vi "Qualify Library Icon Core.vi"(0 "VI Reference":refnum<vi>, 11 "error in":errorcluster) -> (3 "Class?":bool, 4 "Good Library Icon":bool, 6 "Maximum Number of Rows":i32, 8 "Library Path":path, 10 "Number of Rows in Icon":i32, 14 "Icon Image":picture, 15 "error out":errorcluster)   [LabVIEW 2025, in "Text-Based VI Icon.lvlib"]
uses:
  <vilib>/LabVIEW Icon API/Set Text Icon/Text-Based VI Icon.lvlib
panel:
  out "Left and Right Good (for Debugging)":bool
  out "Top and Bottom Good (for Debugging)":bool
  out "Good Frame Color (for Debugging)":bool
  out "Supported Size or Shape (for Debugging)":bool
  out "Last True Mask + 1 (for Debugging)":i32
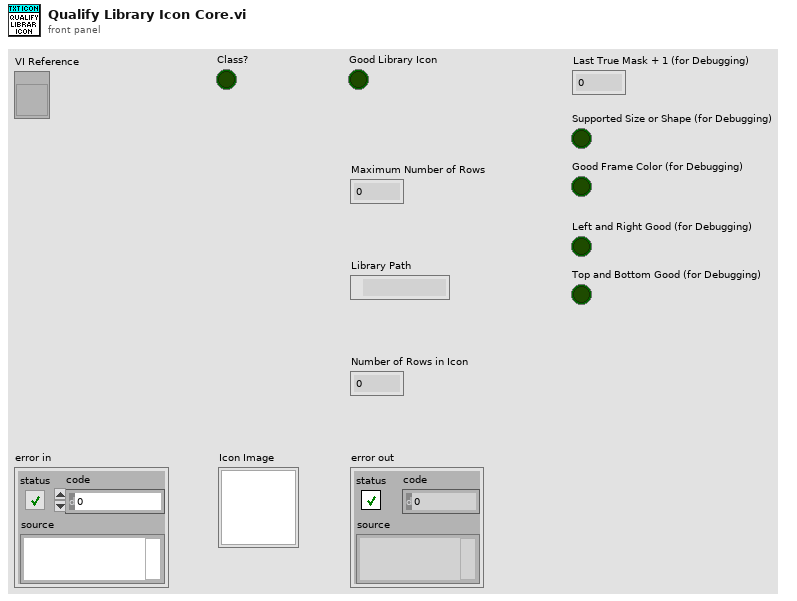
[diagram p1: front panel]
types:
  T1 = typedef "imagedata.ctl" = cluster{"image type":i32, "image depth":i32, "image":u8[], "mask":u8[], "colors":u32[], "Rectangle":cluster{"left":i16, "top":i16, "right":i16, "bottom":i16}}
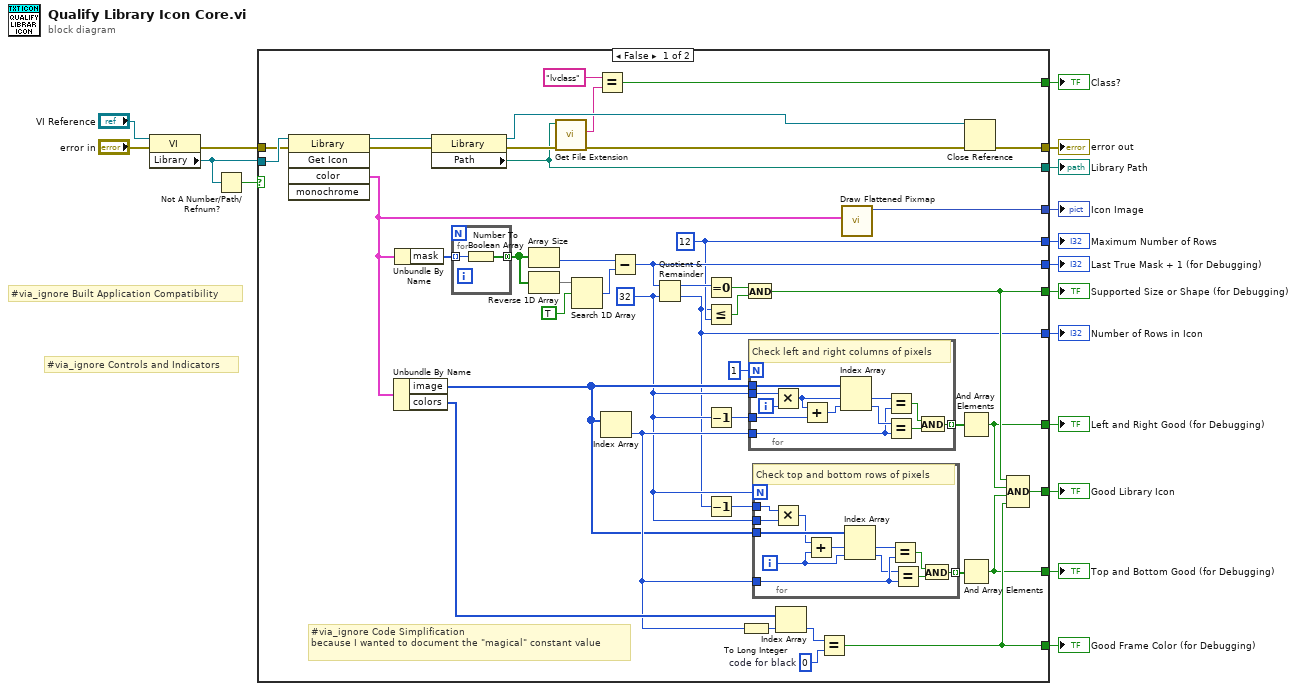
[diagram p0: block diagram]
diagram:
  # "#via_ignore Built Application Compatibility"
  # "#via_ignore Controls and Indicators"
  n1 = property class="VI"(reference="VI Reference", error in="error in") -> (error out=w15:errorcluster, "Library"=w16:refnum<vi>)  [unwired: 1 out]
  n2 = Not A Number/Path/Refnum?(number/path/refnum=w16) -> (NaN/Path/Refnum?=w17:bool)
  n3 = case shown="False" w17 {
    tunnel: w16 -> [w60 _]
    tunnel: w15 -> [w59 w87]
    tunnel: [w28 w87] -> w14
    tunnel: [w49 _] -> w13
    tunnel: [w36 _] -> w12
    tunnel: [w34 _] -> w11
    tunnel: [w33 _] -> w10
    tunnel: [w35 _] -> w9
    tunnel: [w37 _] -> w8
    tunnel: [w32 _] -> w7
    tunnel: [w21 _] -> w6
    tunnel: [w29 _] -> w3
    tunnel: [w22 _] -> w2
    tunnel: [w19 _] -> w1
    frame False {
      w47 = u32 0  # code for black
      w29 = 12 ("y")
      w38 = 32 ("y")
      # "#via_ignore Code Simplification\nbecause I wanted to document the \"magical\" constant value"
      n4 = invoke class="Library" method="Get Icon"(reference=w60, error in=w59) -> (reference out=w31:refnum<vi>, error out=w30:errorcluster, "color"=w20:T1)  [unwired: 3 in, 2 out]
      n5 = Unbundle By Name(w20) -> ("image"=w42:u8[], "colors"=w48:u32[])
      n6 = Unbundle By Name(w20) -> ("mask"=w55:u8[])
      n7 = property class="Library"(reference=w31, error in=w30) -> (reference out=w27:refnum<vi>, error out=w26:errorcluster, "Path"=w21:path)
      n8 = for {
        tunnel: w55 -> [w86] mode=indexing
        tunnel: [w85] -> w52 mode=concatenating
        n9 = Number To Boolean Array(number=w86) -> (Boolean array=w85:bool[])
      }
      n10 = Array Size(array=w52) -> (size(s)=w51:i32)
      n11 = Reverse 1D Array(array=w52) -> (reversed array=w54:bool[])
      n12 = call <vilib>:"Get File Extension.vi"("error in (no error)"=w26, "file"=w21) -> ("error out"=w25:errorcluster, "lowercase file extension"=w24:string)  [unwired: 5 in, 3 out]
      n13 = Search 1D Array(1D array=w54, element=TRUE) -> (index of element=w50:i32)  [unwired: 1 in]
      n14 = Equal?(x="lvclass", y=w24) -> (x = y?=w22:bool)
      n15 = Index Array(array=w42) -> (element=w43:u8)  [unwired: 1 in]
      n16 = Subtract(x=w51, y=w50) -> (x-y=w49:i32)
      n17 = Quotient & Remainder(x=w49, y=w38) -> (x-y*floor(x/y)=w58:i32, floor(x/y)=w19:i32)
      n18 = Equal To 0?(x=w58) -> (x = 0?=w57:bool)
      n19 = Less Or Equal?(x=w19, y=w29) -> (x <= y?=w56:bool)
      n20 = Decrement(x=w38) -> (x-1=w40:i32)
      n21 = Decrement(x=w19) -> (x-1=w44:i32)
      n22 = To Long Integer(number=w43) -> (32bit integer=w46:i32)
      n23 = And(x=w57, y=w56) -> (x .and. y?=w36:bool)
      n24 = for {
        N: 1 -> [_]
        tunnel: w43 -> [w74]
        tunnel: [w82] -> w41 mode=indexing
        tunnel: w40 -> [w80]
        tunnel: w42 -> [w78]
        tunnel: w38 -> [w76]
        i -> [w81]
        # "Check left and right columns of pixels"
        n25 = Multiply(x=w76, y=w81) -> (x*y=w73:i32)
        n26 = Add(x=w73, y=w80) -> (x+y=w75:i32)
        n27 = Index Array(array=w78, index #1=w73, index #2=w75) -> (element #1=w77:u8, element #2=w79:u8)
        n28 = Equal?(x=w77, y=w74) -> (x = y?=w84:bool)
        n29 = Equal?(x=w79, y=w74) -> (x = y?=w83:bool)
        n30 = And(x=w84, y=w83) -> (x .and. y?=w82:bool)
      }
      n31 = for {
        N: w38 -> [_]
        tunnel: w42 -> [w72]
        tunnel: w44 -> [w71]
        tunnel: w43 -> [w66]
        tunnel: [w62] -> w45 mode=indexing
        tunnel: w38 -> [w61]
        i -> [w68]
        # "Check top and bottom rows of pixels"
        n32 = Multiply(x=w71, y=w61) -> (x*y=w70:i32)
        n33 = Add(x=w70, y=w68) -> (x+y=w69:i32)
        n34 = Index Array(array=w72, index #1=w69, index #2=w68) -> (element #1=w67:u8, element #2=w65:u8)
        n35 = Equal?(x=w67, y=w66) -> (x = y?=w64:bool)
        n36 = Equal?(x=w65, y=w66) -> (x = y?=w63:bool)
        n37 = And(x=w64, y=w63) -> (x .and. y?=w62:bool)
      }
      n38 = Index Array(array=w48, index=w46) -> (element=w39:u32)
      n39 = Equal?(x=w39, y=w47) -> (x = y?=w34:bool)
      n40 = call <vilib>:"Draw Flattened Pixmap.vi"("image data"=w20) -> ("new picture"=w37:picture)  [unwired: 8 in]
      n41 = And Array Elements(Boolean array=w41) -> (logical AND=w35:bool)
      n42 = And Array Elements(Boolean array=w45) -> (logical AND=w33:bool)
      n43 = Close Reference(reference=w27, error in (no error)=w25) -> (error out=w28:errorcluster)
      n44 = Compound Arithmetic op=AND(w36, w35, w33, w34) -> (w32:bool)
    }
    frame True {
    }
  }
  "error out" <- w14
  "Last True Mask + 1 (for Debugging)" <- w13
  "Supported Size or Shape (for Debugging)" <- w12
  "Good Frame Color (for Debugging)" <- w11
  "Top and Bottom Good (for Debugging)" <- w10
  "Left and Right Good (for Debugging)" <- w9
  "Icon Image" <- w8
  "Good Library Icon" <- w7
  "Library Path" <- w6
  "Maximum Number of Rows" <- w3
  "Class?" <- w2
  "Number of Rows in Icon" <- w1
